vi "labview_tcp_client.vi"() -> ()   [LabVIEW 2018]
doc: "You can use the System Exec VI to call command line utilities that return standard output to the command shell. You also can call interactive applications that you intend to launch using System Exec, but interact with using the UI of the executable."
panel:
  out "data out":string
  in  "Stop Button":bool
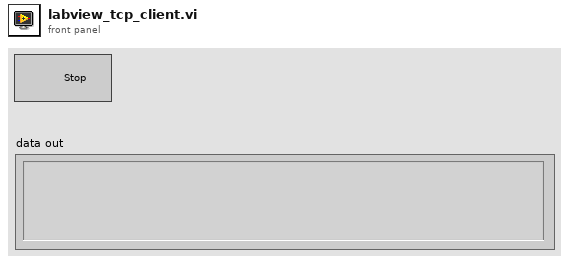
[diagram p1: front panel]
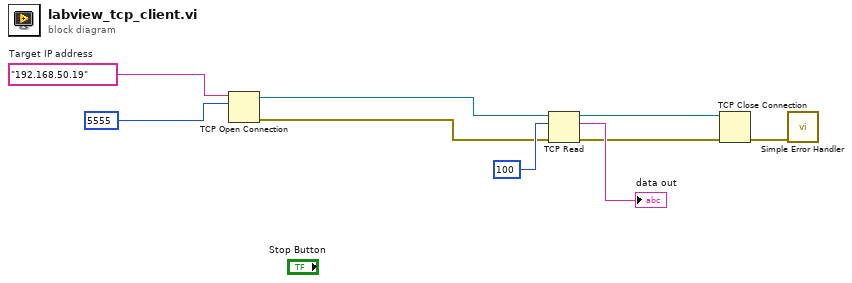
[diagram p0: block diagram]
diagram:
  w9 = "192.168.50.19"  # Target IP address
  n1 = TCP Open Connection(address=w9, remote port or service name=5555) -> (connection ID=w2:refnum<k5>, error out=w1:errorcluster)  [unwired: 3 in]
  n2 = TCP Read(connection ID=w2, bytes to read=100, error in (no error)=w1) -> (connection ID out=w4:refnum<k5>, data out=→"data out":string, error out=w5:errorcluster)  [unwired: 2 in]
  n3 = TCP Close Connection(connection ID=w4, error in (no error)=w5) -> (error out=w3:errorcluster)  [unwired: 1 in, 1 out]
  n4 = call <vilib>:"Simple Error Handler.vi"("error in (no error)"=w3) -> ()  [unwired: 2 in, 7 out]
